vi "Finish.vi"   [LabVIEW 2015]
doc: "This VI is called just before exiting. It is expected to close I/O refnum, save collected data, etc."
uses:
  <vilib>/Rock Robotics/WPI/Utilities/WPI_GetSetVariantRefNum.vi
  NavX/navX Library v2.lvlib
types:
  T1 = typedef "navX Library v2.lvlib/Z900_navX_DeviceTypeDef.ctl" = cluster{"Interface":cluster{"Protocol":T2, "Update Rate (4Hz-60Hz)":u8, "navX Open TypeDef":variant}, "Notify Packet":refnum<notifier>, "Loop VI Refnum":refnum<vi>, "Ready to Close Occurrence Refnum":refnum<k4>}
  T2 = typedef "navX Library v2.lvlib/Z900_navX_ProtocolTypeDef.ctl" = enum16{"SERIAL", "I2C", "SPI"}
  T3 = typedef "WPI_JoystickDevRef.ctl" = cluster{"Device":T4}
  T4 = typedef "WPI_JoystickDeviceEnum.ctl" = enum16{"USB 0", "USB 1", "USB 2", "USB 3", "USB 4", "USB 5"}
  T5 = typedef "WPI_RobotDriveDevRef.ctl" = cluster{"DevStatus":errorcluster, "Motors[]":T6[], "Square Inputs":bool, "Max Output":dbl}
  T6 = typedef "WPI_MotorControlDeviceRef.ctl" = cluster{"DeviceStatus":errorcluster, "Type":T7, "PWM":cluster{"PWM Channel":T8, "DeadBand":T9}, "CAN":cluster{"Device Number":u8, "Control Mode":T10, "Semaphore":T11, "Max Vout":dbl, "TalonSRX Control Mode":T12}, "Invert":bool}
  T7 = typedef "WPI_MotorControlType.ctl" = enum16{"PWM", "CAN", "CANTalonSRX"}
  T8 = typedef "FPGA_DIOPWMChannel.ctl" = enum8{"PWM 0", "PWM 1", "PWM 2", "PWM 3", "PWM 4", "PWM 5", "PWM 6", "PWM 7", "PWM 8", "PWM 9", "PWM MXP 0", "PWM MXP 1", "PWM MXP 2", "PWM MXP 3", "PWM MXP 4", "PWM MXP 5", "PWM MXP 6", "PWM MXP 7", "PWM MXP 8", "PWM MXP 9", "Invalid"}
  T9 = typedef "WPI_PWMDeadband.ctl" = cluster{"Name":string, "maxPositivePwm":i32, "minPositivePwm":i32, "centerPwm":i32, "maxNegativePwm":i32, "minNegativePwm":i32, "angularRange":u16}
  T10 = typedef "WPI_CANJaguar_ControlMode.ctl" = enum8{"Percent VBus", "Current", "Speed", "Position", "Voltage"}
  T11 = typedef "Semaphore RefNum" = refnum<k1>
  T12 = typedef "WPI_CANTalonSRX_APIControlMode.ctl" = enum8{"Percent VBus", "Speed", "Position", "Slave", "Unchanged / Invalid", "Voltage Compensation", "Current", "Motion Profile"}
  T13 = typedef "WPI_PotentiometerDevRef.ctl" = cluster{"DevStatus":errorcluster, "Analog Channel":T14, "Invert Output":bool}
  T14 = typedef "FPGA_AIChannel.ctl" = enum8{"AI 0", "AI 1", "AI 2", "AI 3", "AI MXP 0", "AI MXP 1", "AI MXP 2", "AI MXP 3", "Invalid"}
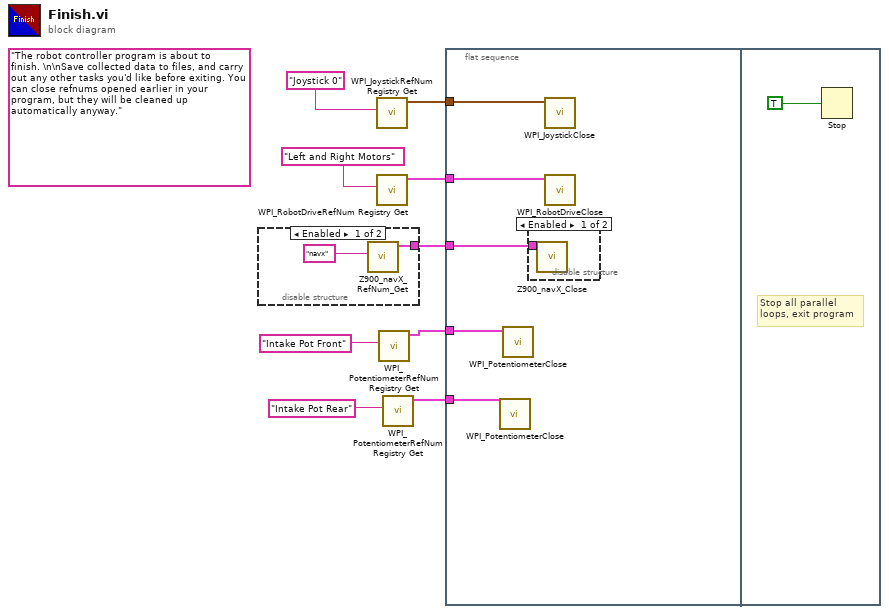
[diagram p0: block diagram]
diagram:
  (unwired) "The robot controller program is about to finish. \n\nSave collected data to files, and carry out any other tasks you'd like before exiting. You can close refnums opened earlier in your program, but they will be cleaned up automatically anyway."
  n1 = disable-structure shown="Enabled" {
    disable-tunnel: [w10 _] -> w5
    frame Enabled {
      n2 = call "Z900_navX_RefNum_Get.vi"("refnum name"="navx") -> ("navX Device"=w10:T1)  [unwired: 9 in, 1 out]
    }
    frame Disabled {
    }
  }
  n3 = call <vilib>:"WPI_JoystickRefNum Registry Get.vi"("refnum name"="Joystick 0") -> ("JoystickDevRef"=w6:T3)  [unwired: 1 in, 9 out]
  n4 = call <vilib>:"WPI_RobotDriveRefNum Registry Get.vi"("refnum name"="Left and Right Motors") -> ("RobotDriveDevRef"=w7:T5)  [unwired: 1 in, 9 out]
  n5 = call <vilib>:"WPI_PotentiometerRefNum Registry Get.vi"("refnum name"="Intake Pot Front") -> ("PotDevRef"=w4:T13)  [unwired: 9 in, 1 out]
  n6 = call <vilib>:"WPI_PotentiometerRefNum Registry Get.vi"("refnum name"="Intake Pot Rear") -> ("PotDevRef"=w1:T13)  [unwired: 9 in, 1 out]
  n7 = flat-sequence {
    tunnel: w7 -> [w16]
    tunnel: w6 -> [w15]
    tunnel: w5 -> [w14]
    tunnel: w4 -> [w13]
    tunnel: w1 -> [w12]
    frame #0 {
      n8 = call <vilib>:"WPI_PotentiometerClose.vi"("PotDevRef"=w12) -> ()  [unwired: 10 in, 1 out]
      n9 = call <vilib>:"WPI_PotentiometerClose.vi"("PotDevRef"=w13) -> ()  [unwired: 10 in, 1 out]
      n10 = disable-structure shown="Enabled" {
        disable-tunnel: w14 -> [w17 _]
        frame Enabled {
          n11 = call "Z900_navX_Close.vi"("navX Device"=w17) -> ()  [unwired: 10 in, 1 out]
        }
        frame Disabled {
        }
      }
      n12 = call <vilib>:"WPI_JoystickClose.vi"("JoystickDevRef"=w15) -> ()  [unwired: 11 out]
      n13 = call <vilib>:"WPI_RobotDriveClose.vi"("RobotDriveDevRef"=w16) -> ()  [unwired: 1 in, 10 out]
    }
    frame #1 {
      # "Stop all parallel\nloops, exit program"
      n14 = Stop(stop? (T)=TRUE ("Quit")) -> ()
    }
  }
